vi "show_run_time(SubVI).vi"(11 "String":string) -> ()   [LabVIEW 2015]
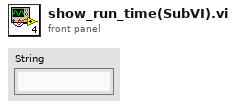
[diagram p1: front panel]
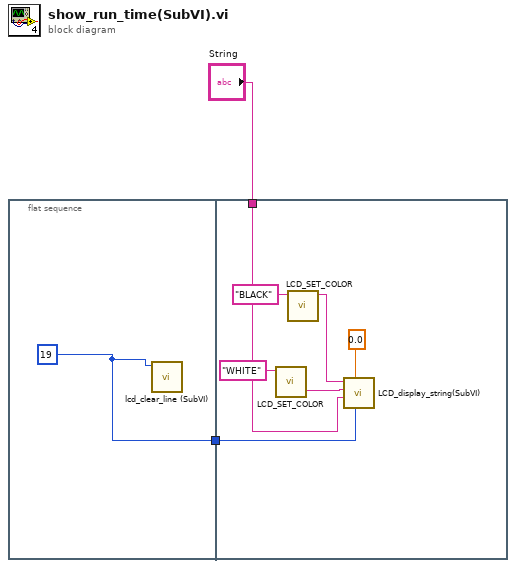
[diagram p0: block diagram]
diagram:
  n1 = flat-sequence {
    tunnel: [w3] -> w2
    tunnel: w2 -> [w10]
    tunnel: "String" -> [w6]
    frame #0 {
      w3 = 19
      n2 = call "lcd_clear_line (SubVI).vi"("Numeric"=w3) -> ()  [unwired: 11 in]
    }
    frame #1 {
      n3 = call "LCD_SET_COLOR.vi"("String in"="WHITE") -> ("String out"=w8:string)  [unwired: 10 in]
      n4 = call "LCD_SET_COLOR.vi"("String in"="BLACK") -> ("String out"=w7:string)  [unwired: 10 in]
      n5 = call "LCD_display_string(SubVI).vi"("y"=w10, "x"=0.0, "String"=w6, "char_color"=w8, "background"=w7) -> ()  [unwired: 7 in]
    }
  }
